vi "Convert_PathWeaverJSON_To_TrajectoryFile.vi"() -> ()   [LabVIEW 2019]
uses:
  <vilib>/Rock Robotics/WPI/ThirdParty/JAS_Junk/TrajLib/TRAJ_STATE.ctl
  <vilib>/Rock Robotics/WPI/ThirdParty/JAS_Junk/TrajLib/POSE2D.ctl
  <vilib>/Rock Robotics/WPI/ThirdParty/JAS_Junk/TrajLib/TRANSLATION2D.ctl
  <vilib>/Rock Robotics/WPI/ThirdParty/JAS_Junk/TrajLib/ROTATION2D.ctl
  <vilib>/Rock Robotics/WPI/ThirdParty/JAS_Junk/TrajLib/DISPLAY_WAYPOINT.ctl
  <vilib>/Rock Robotics/WPI/ThirdParty/JAS_Junk/TrajLib/Trajectory_Library.lvlib
panel:
  in  "End Program":bool
  in  "Tab Control":T1(tab)
  in  "Convert upper left \norigin to lower left":bool
  in  "PathWeaver JSON File":path
  in  "Read JSON Fiile":bool
  out "File Read Error":errorcluster
  in  "PathWeaver Length Units":T2(radio)
  in  "WheelBase":dbl=0.6
  out "Position":cluster{dbl[], dbl[]}[](graph)
  out "Trajectory Data":cluster{dbl[], dbl[]}[](graph)
  out "Traj States\nSize":i32
  out "Trajectory States":T3[](array[typedef]) {"POSE"."ROTATION"."SIN" format="%13.4f"; "POSE"."ROTATION"."COS" format="%13.4f"; "POSE"."ROTATION"."VALUE" format="%13.4f"; "POSE"."TRANSLATION"."Y" format="%14.3f"; "POSE"."TRANSLATION"."X" format="%14.3f"}
  out "File Saved\nWithout\nError":bool
  in  "Trajectory Type":enum32{"Radio Selection 1", "Radio Selection 2"}(radio)
  out "File Creation\nError":errorcluster
  in  "Trajectory File Comment":string
  in  "Trajectory File Name":path
  in  "CreateCmdList":bool
  out "Ready to\nWrite FIle":bool
  # "Convert Pathweaver JSON file to trajectory file"
  # "Instructions: \n---------------- \nThis utility reads a JSON file create from PathWeaver.  The results are plotted for review.  This file can then be written to a Trajectory Library CSV file.\n\nNotes:\n---------\n - Pathweaver sets the Y orign at the top left.  This trajectory library utilties use the bottom right.  This utility converts the Y position value to be consistent. \n   There are no consequences when the trajectory is saved as a robot relative trajectory.  For absolute trajectories, the robot position needs to\n   condier this."
  # "Meters"
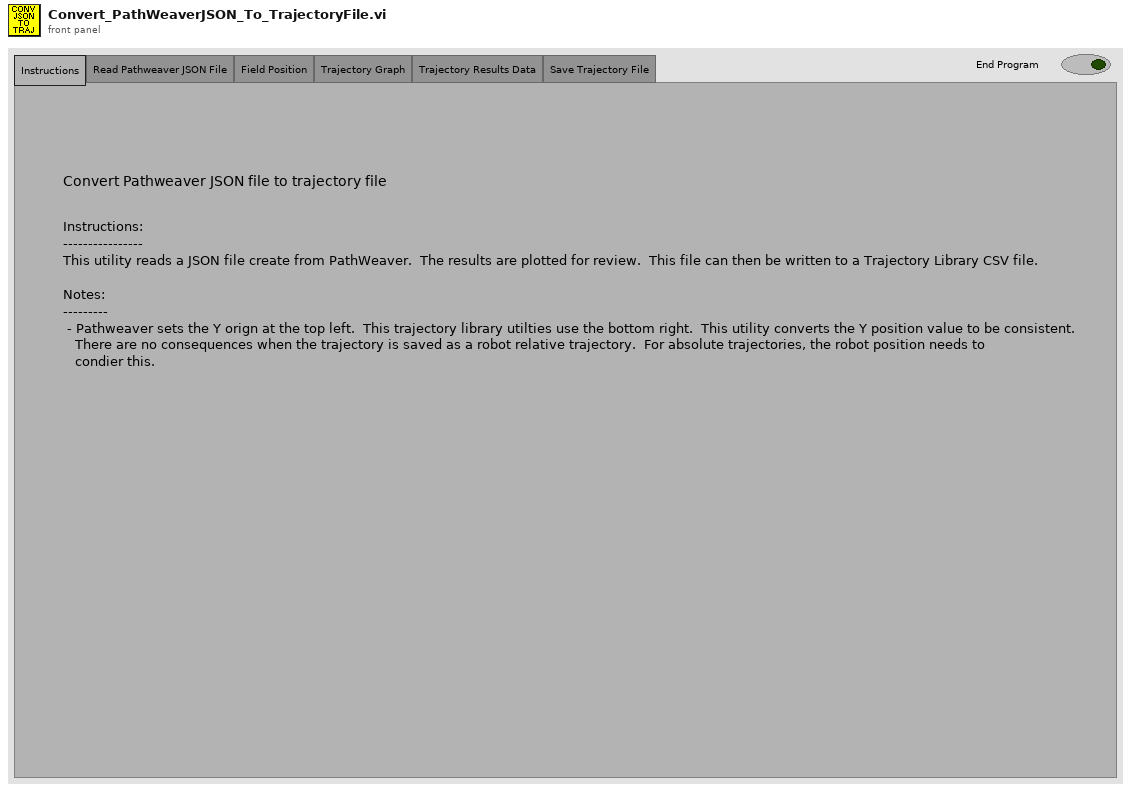
[diagram p1: front panel]
types:
  T1 = enum32{"Instructions", "Read Pathweaver JSON File", "Field Position", "Trajectory Graph", "Trajectory Results Data", "Save Trajectory File"}
  T2 = enum32{"Radio Selection 1", "Radio Selection 2", "Radio Selection 3", "Radio Selection 4", "Radio Selection 5"}
  T3 = typedef "Trajectory_Library.lvlib/TRAJ_STATE.ctl" = cluster{"TimeSeconds":dbl, "Velocity":dbl, "Acceleration":dbl, "POSE":T4, "Curvature":dbl}
  T4 = typedef "Trajectory_Library.lvlib/POSE2D.ctl" = cluster{"TRANSLATION":T5, "ROTATION":T6}
  T5 = typedef "Trajectory_Library.lvlib/TRANSLATION2D.ctl" = cluster{"X":dbl, "Y":dbl}
  T6 = typedef "Trajectory_Library.lvlib/ROTATION2D.ctl" = cluster{"VALUE":dbl, "COS":dbl, "SIN":dbl}
  T7 = typedef "Trajectory_Library.lvlib/DISPLAY_WAYPOINT.ctl" = cluster{"X":dbl, "Y":dbl, "ANGLE":dbl}
  T8 = typedef "Trajectory_Library.lvlib/TRAJECTORY.ctl" = cluster{"TotalTImeSecs":dbl, "States":T3[]}
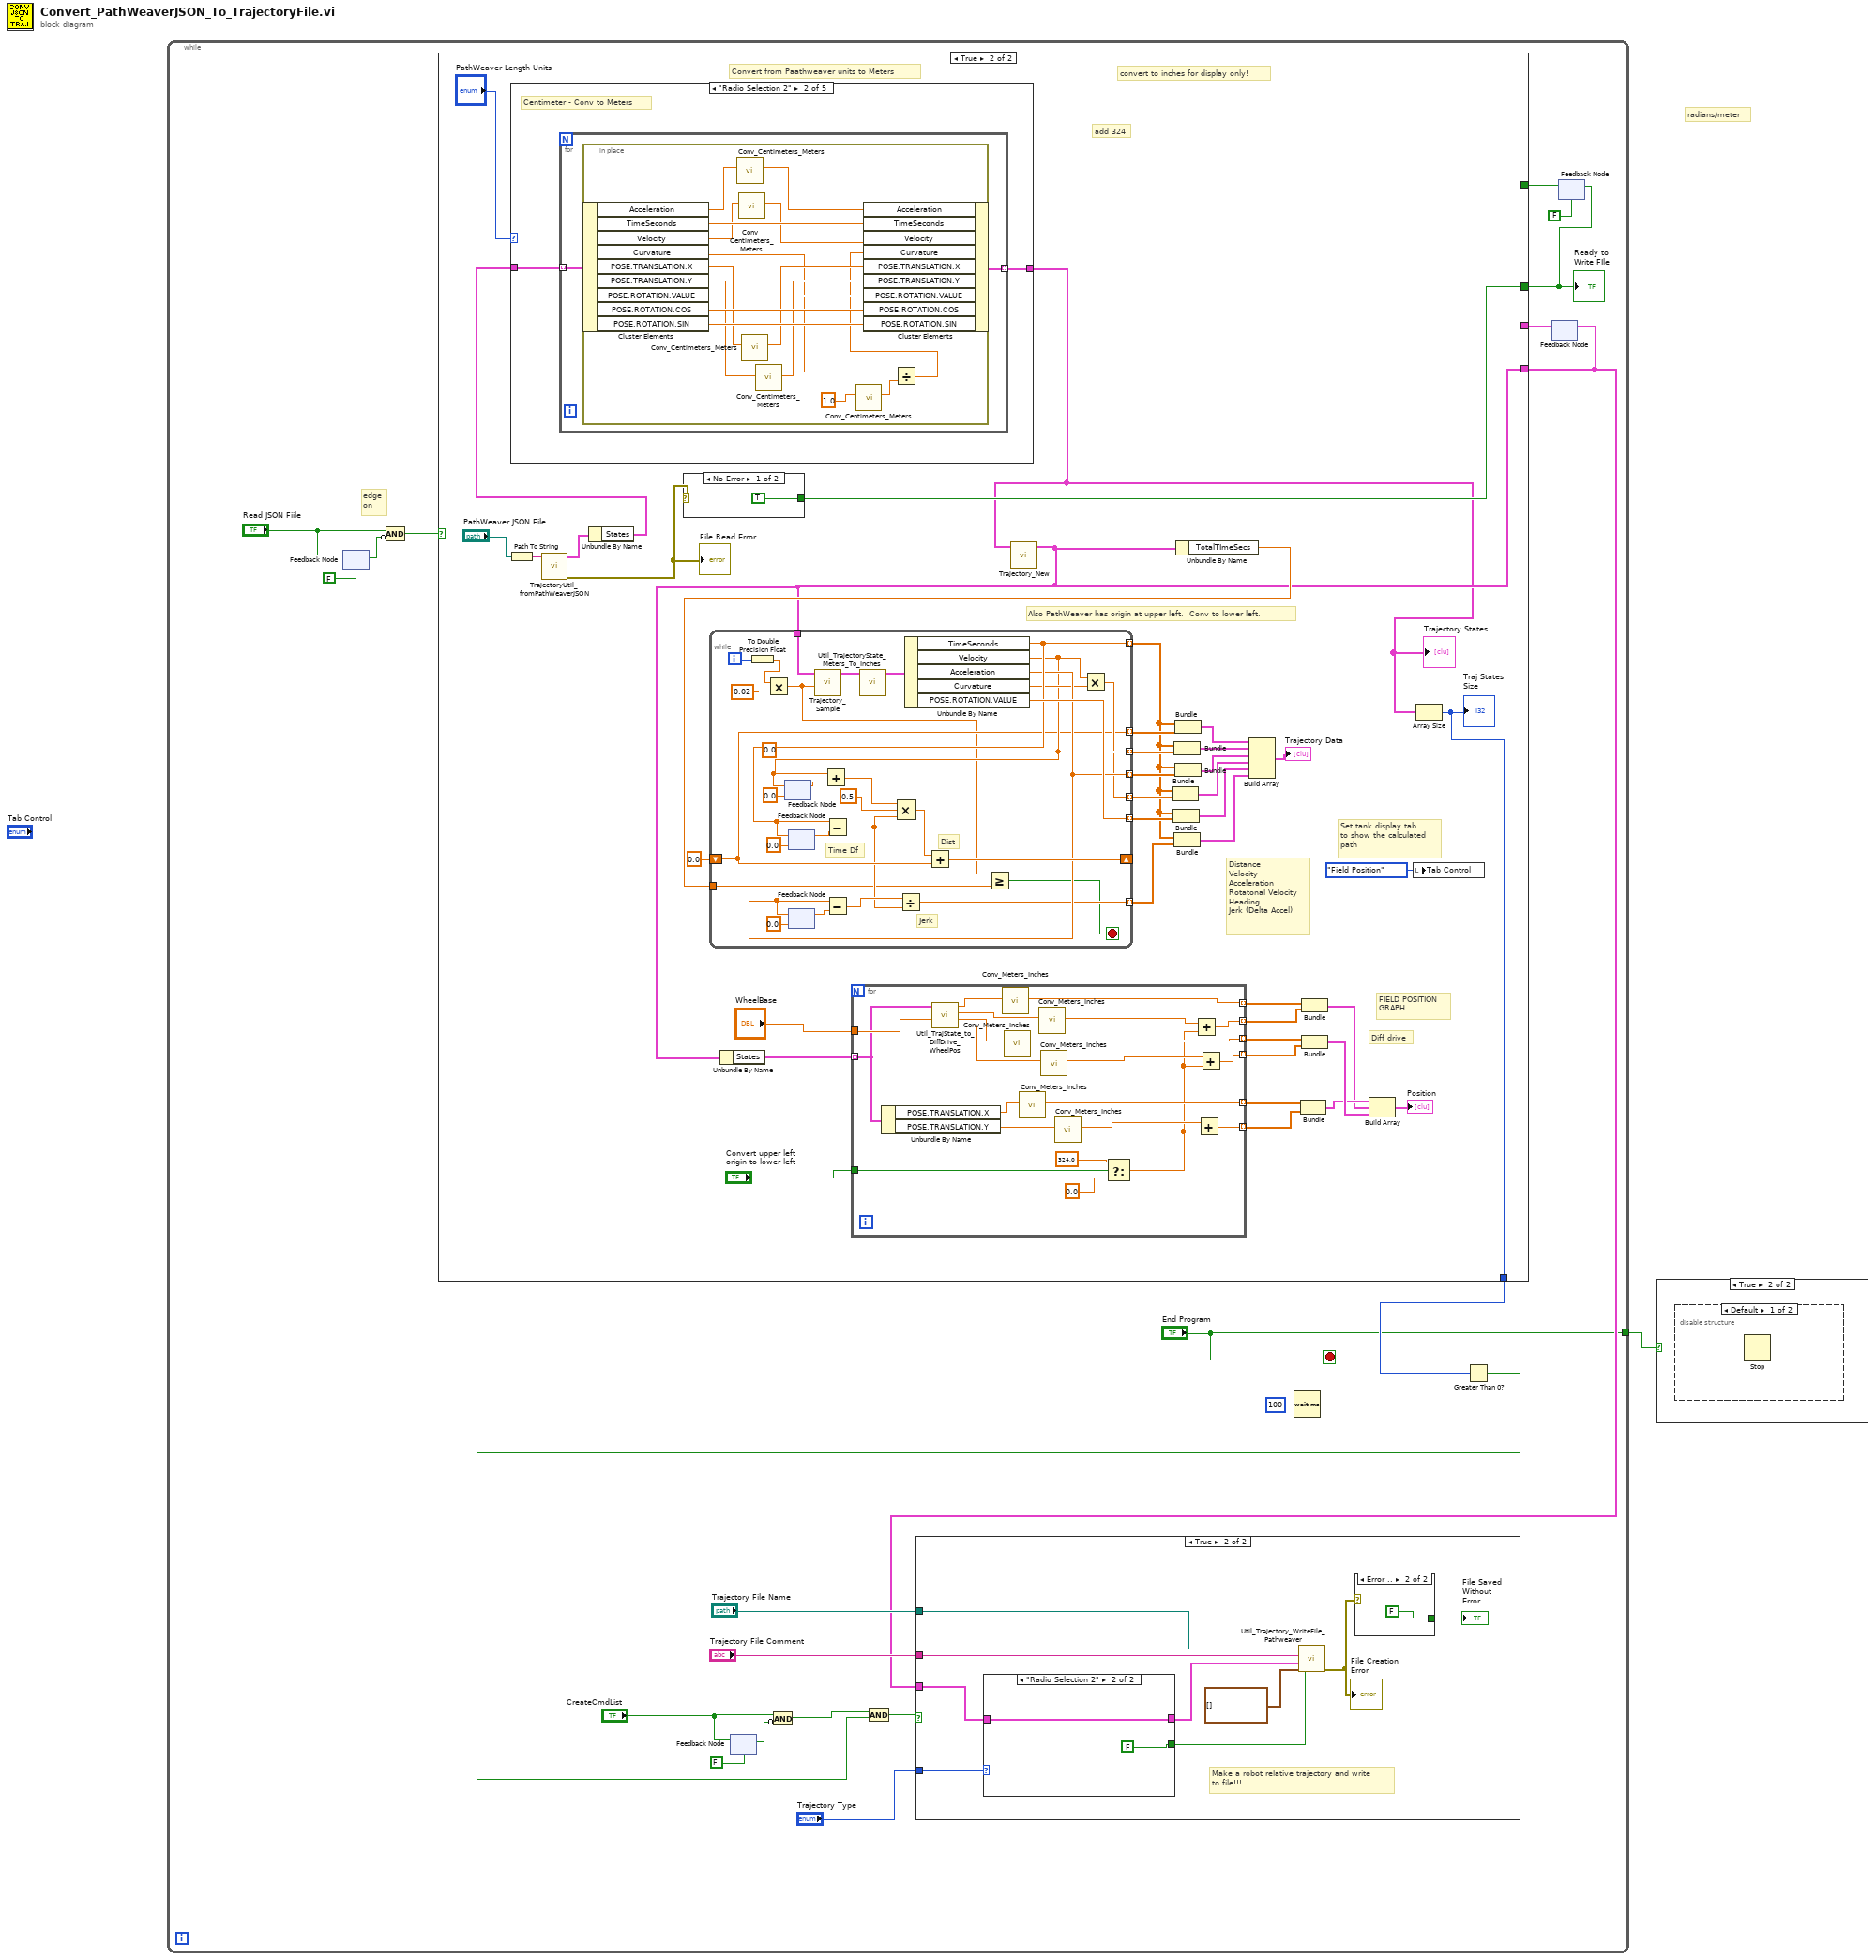
[diagram p0: block diagram]
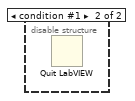
[diagram p3: hidden frame]
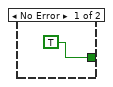
[diagram p5: hidden frame]
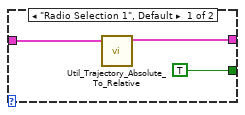
[diagram p6: hidden frame]
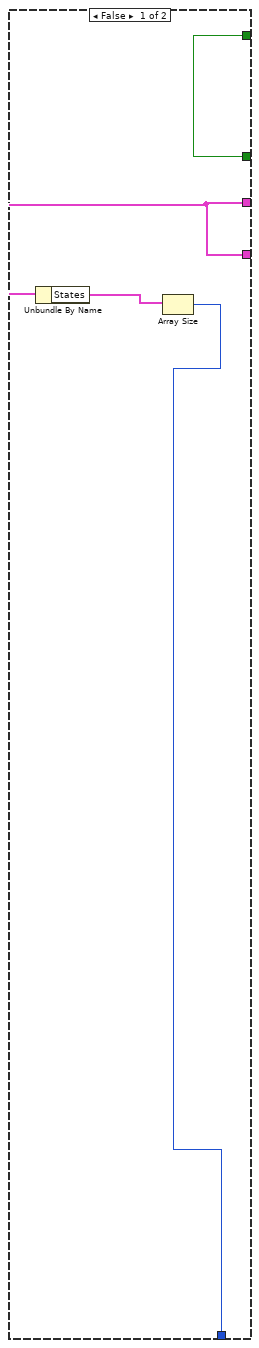
[diagram p7: hidden frame]
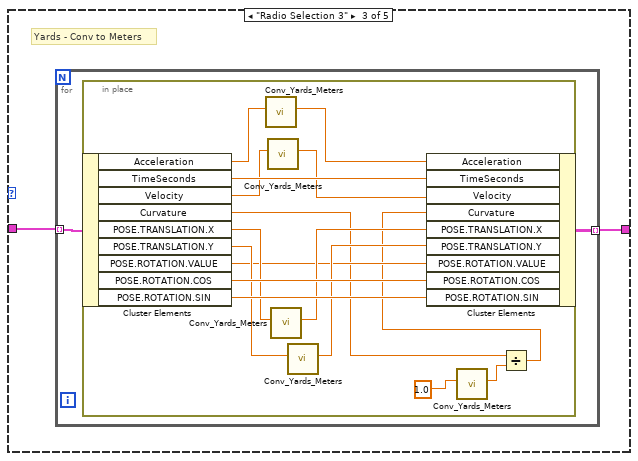
[diagram p9: hidden frame]
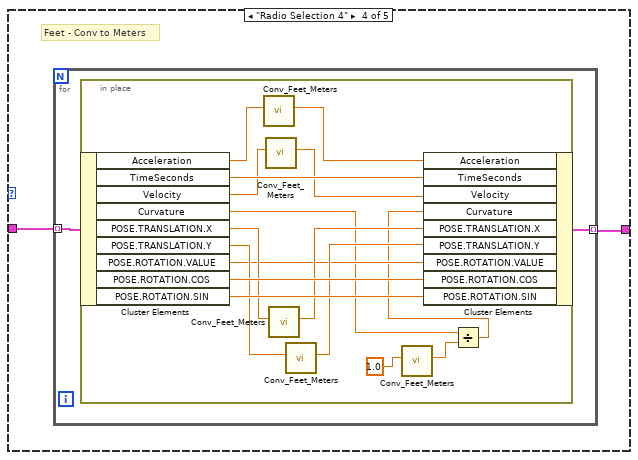
[diagram p10: hidden frame]
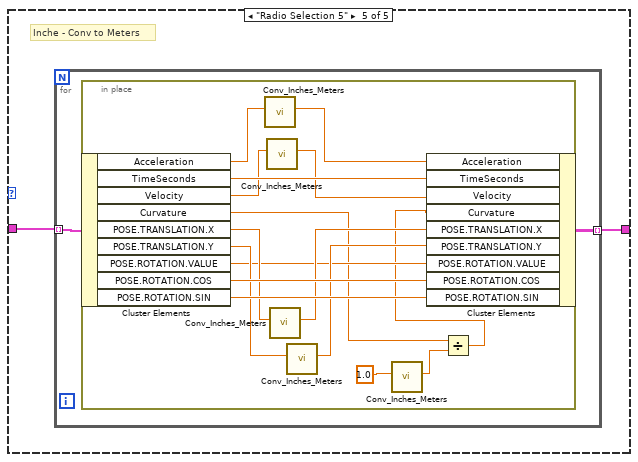
[diagram p11: hidden frame]
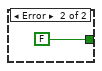
[diagram p12: hidden frame]
diagram:
  # "radians/meter"
  n1 = while {
    tunnel: ["End Program"] -> w1
    stop <- "End Program" stop-if-true
    # "edge\non"
    n2 = feedback #1(FALSE ("CreateCmdList")) -> (w11:bool)
    n3 = feedback-in #1("Read JSON Fiile") -> ()
    n4 = Compound Arithmetic op=AND("Read JSON Fiile", invert w11) -> (w9:bool)
    n5 = feedback-in #2("CreateCmdList") -> ()
    n6 = feedback #2(FALSE ("CreateCmdList")) -> (w14:bool)
    n7 = Compound Arithmetic op=AND("CreateCmdList", invert w14) -> (w13:bool)
    n8 = Wait (ms)(milliseconds to wait=u32 100) -> ()  [unwired: 1 out]
    n9 = feedback #3() -> (w21:T8)  [unwired: 1 in]
    n10 = feedback #4(FALSE) -> (w5:bool)
    n11 = case shown="True" w9 {
      tunnel: [w40 w47] -> w17
      tunnel: w21 -> [w40 _]
      tunnel: [w42 w82] -> w16
      tunnel: [w41 w78] -> w7
      tunnel: w5 -> [w41 _]
      frame False {
        n12 = Unbundle By Name(w40) -> ("States"=w39:T3[])
        n13 = Array Size(array=w39) -> (size(s)=w42:i32)
      }
      frame True {
        (unwired) 0.0
        # "add 324"
        # "Diff drive"
        # "FIELD POSITION\nGRAPH"
        # "Distance\nVelocity\nAcceleration\nRotatonal Velocity\nHeading\nJerk (Delta Accel)"
        # "Also PathWeaver has origin at upper left.  Conv to lower left."
        # "convert to inches for display only!"
        # "Convert from Paathweaver units to Meters"
        # "Set tank display tab\nto show the calculated\npath"
        n14 = Path To String(path="PathWeaver JSON File") -> (string=w81:string)
        n15 = call <vilib>:"TrajectoryUtil_fromPathWeaverJSON.vi"("FileName"=w81) -> ("error out"=w79:errorcluster, "outTRAJECTORY"=w76:T8)  [unwired: 8 in, 1 out]
        "File Read Error" <- w79
        n16 = Unbundle By Name(w76) -> ("States"=w75:T3[])
        n17 = case shown="\"Radio Selection 2\"" "PathWeaver Length Units" {
          tunnel: w75 -> [w133 w134 w155 w175 w195]
          tunnel: [w133 w135 w154 w174 w194] -> w44
          frame "Radio Selection 1" {
            # "Meters - do nothing"
          }
          frame "Radio Selection 2" {
            # "Centimeter - Conv to Meters"
            n18 = for {
              tunnel: w134 -> [w137] mode=indexing
              tunnel: [w136] -> w135 mode=indexing
              n19 = in-place {
                n20 = in-place-cluster #5(w137) -> ("Acceleration"=w145:dbl, "TimeSeconds"=w153:dbl, "Velocity"=w147:dbl, "Curvature"=w138:dbl, "POSE.TRANSLATION.X"=w149:dbl, "POSE.TRANSLATION.Y"=w150:dbl, "POSE.ROTATION.VALUE"=w142:dbl, "POSE.ROTATION.COS"=w152:dbl, "POSE.ROTATION.SIN"=w151:dbl)
                n21 = call <vilib>:"Conv_Centimeters_Meters.vi"("Centimeter"=w145) -> ("Meters"=w144:dbl)  [unwired: 10 in]
                n22 = call <vilib>:"Conv_Centimeters_Meters.vi"("Centimeter"=w147) -> ("Meters"=w146:dbl)  [unwired: 10 in]
                n23 = call <vilib>:"Conv_Centimeters_Meters.vi"("Centimeter"=w149) -> ("Meters"=w148:dbl)  [unwired: 10 in]
                n24 = call <vilib>:"Conv_Centimeters_Meters.vi"("Centimeter"=w150) -> ("Meters"=w143:dbl)  [unwired: 10 in]
                n25 = call <vilib>:"Conv_Centimeters_Meters.vi"("Centimeter"=1.0) -> ("Meters"=w139:dbl)  [unwired: 10 in]
                n26 = Divide(x=w138, y=w139) -> (x/y=w141:dbl)
                n27 = in-place-cluster #5("Acceleration"=w144, "TimeSeconds"=w153, "Velocity"=w146, "Curvature"=w141, "POSE.TRANSLATION.X"=w148, "POSE.TRANSLATION.Y"=w143, "POSE.ROTATION.VALUE"=w142, "POSE.ROTATION.COS"=w152, "POSE.ROTATION.SIN"=w151) -> (w136:T3)
              }
            }
          }
          frame "Radio Selection 3" {
            # "Yards - Conv to Meters"
            n28 = for {
              tunnel: w155 -> [w157] mode=indexing
              tunnel: [w156] -> w154 mode=indexing
              n29 = in-place {
                n30 = in-place-cluster #6(w157) -> ("Acceleration"=w165:dbl, "TimeSeconds"=w173:dbl, "Velocity"=w167:dbl, "Curvature"=w161:dbl, "POSE.TRANSLATION.X"=w169:dbl, "POSE.TRANSLATION.Y"=w170:dbl, "POSE.ROTATION.VALUE"=w162:dbl, "POSE.ROTATION.COS"=w172:dbl, "POSE.ROTATION.SIN"=w171:dbl)
                n31 = call <vilib>:"Conv_Yards_Meters.vi"("Yards"=w165) -> ("Meters"=w164:dbl)  [unwired: 10 in]
                n32 = call <vilib>:"Conv_Yards_Meters.vi"("Yards"=w167) -> ("Meters"=w166:dbl)  [unwired: 10 in]
                n33 = call <vilib>:"Conv_Yards_Meters.vi"("Yards"=w169) -> ("Meters"=w168:dbl)  [unwired: 10 in]
                n34 = call <vilib>:"Conv_Yards_Meters.vi"("Yards"=w170) -> ("Meters"=w163:dbl)  [unwired: 10 in]
                n35 = call <vilib>:"Conv_Yards_Meters.vi"("Yards"=1.0 ("Centimeter")) -> ("Meters"=w159:dbl)  [unwired: 10 in]
                n36 = Divide(x=w161, y=w159) -> (x/y=w160:dbl)
                n37 = in-place-cluster #6("Acceleration"=w164, "TimeSeconds"=w173, "Velocity"=w166, "Curvature"=w160, "POSE.TRANSLATION.X"=w168, "POSE.TRANSLATION.Y"=w163, "POSE.ROTATION.VALUE"=w162, "POSE.ROTATION.COS"=w172, "POSE.ROTATION.SIN"=w171) -> (w156:T3)
              }
            }
          }
          frame "Radio Selection 4" {
            # "Feet - Conv to Meters"
            n38 = for {
              tunnel: w175 -> [w177] mode=indexing
              tunnel: [w176] -> w174 mode=indexing
              n39 = in-place {
                n40 = in-place-cluster #7(w177) -> ("Acceleration"=w185:dbl, "TimeSeconds"=w193:dbl, "Velocity"=w187:dbl, "Curvature"=w179:dbl, "POSE.TRANSLATION.X"=w189:dbl, "POSE.TRANSLATION.Y"=w190:dbl, "POSE.ROTATION.VALUE"=w182:dbl, "POSE.ROTATION.COS"=w192:dbl, "POSE.ROTATION.SIN"=w191:dbl)
                n41 = call <vilib>:"Conv_Feet_Meters.vi"("Feet"=w185) -> ("Meters"=w184:dbl)  [unwired: 10 in]
                n42 = call <vilib>:"Conv_Feet_Meters.vi"("Feet"=w187) -> ("Meters"=w186:dbl)  [unwired: 10 in]
                n43 = call <vilib>:"Conv_Feet_Meters.vi"("Feet"=w189) -> ("Meters"=w188:dbl)  [unwired: 10 in]
                n44 = call <vilib>:"Conv_Feet_Meters.vi"("Feet"=w190) -> ("Meters"=w183:dbl)  [unwired: 10 in]
                n45 = call <vilib>:"Conv_Feet_Meters.vi"("Feet"=1.0 ("Centimeter")) -> ("Meters"=w180:dbl)  [unwired: 10 in]
                n46 = Divide(x=w179, y=w180) -> (x/y=w178:dbl)
                n47 = in-place-cluster #7("Acceleration"=w184, "TimeSeconds"=w193, "Velocity"=w186, "Curvature"=w178, "POSE.TRANSLATION.X"=w188, "POSE.TRANSLATION.Y"=w183, "POSE.ROTATION.VALUE"=w182, "POSE.ROTATION.COS"=w192, "POSE.ROTATION.SIN"=w191) -> (w176:T3)
              }
            }
          }
          frame "Radio Selection 5" {
            # "Inche - Conv to Meters"
            n48 = for {
              tunnel: w195 -> [w197] mode=indexing
              tunnel: [w196] -> w194 mode=indexing
              n49 = in-place {
                n50 = in-place-cluster #8(w197) -> ("Acceleration"=w205:dbl, "TimeSeconds"=w213:dbl, "Velocity"=w207:dbl, "Curvature"=w199:dbl, "POSE.TRANSLATION.X"=w209:dbl, "POSE.TRANSLATION.Y"=w210:dbl, "POSE.ROTATION.VALUE"=w202:dbl, "POSE.ROTATION.COS"=w212:dbl, "POSE.ROTATION.SIN"=w211:dbl)
                n51 = call <vilib>:"Conv_Inches_Meters.vi"("INCH"=w205) -> ("Meters"=w204:dbl)  [unwired: 10 in]
                n52 = call <vilib>:"Conv_Inches_Meters.vi"("INCH"=w207) -> ("Meters"=w206:dbl)  [unwired: 10 in]
                n53 = call <vilib>:"Conv_Inches_Meters.vi"("INCH"=w209) -> ("Meters"=w208:dbl)  [unwired: 10 in]
                n54 = call <vilib>:"Conv_Inches_Meters.vi"("INCH"=w210) -> ("Meters"=w203:dbl)  [unwired: 10 in]
                n55 = call <vilib>:"Conv_Inches_Meters.vi"("INCH"=1.0 ("Centimeter")) -> ("Meters"=w200:dbl)  [unwired: 10 in]
                n56 = Divide(x=w199, y=w200) -> (x/y=w198:dbl)
                n57 = in-place-cluster #8("Acceleration"=w204, "TimeSeconds"=w213, "Velocity"=w206, "Curvature"=w198, "POSE.TRANSLATION.X"=w208, "POSE.TRANSLATION.Y"=w203, "POSE.ROTATION.VALUE"=w202, "POSE.ROTATION.COS"=w212, "POSE.ROTATION.SIN"=w211) -> (w196:T3)
              }
            }
          }
        }
        "Trajectory States" <- w44
        n58 = case shown="No Error" w79 {
          tunnel: [TRUE FALSE] -> w78
          frame No Error {
          }
          frame Error {
          }
        }
        n59 = call <vilib>:"Trajectory_New.vi"("TRAJ_STATES"=w44) -> ("TRAJECTORY"=w47:T8)  [unwired: 10 in]
        n60 = Unbundle By Name(w47) -> ("States"=w46:T3[])
        n61 = for {
          tunnel: w46 -> [w98] mode=indexing
          tunnel: "WheelBase" -> [w103]
          tunnel: [w93] -> w56 mode=indexing
          tunnel: [w95] -> w55 mode=indexing
          tunnel: [w91] -> w54 mode=indexing
          tunnel: [w94] -> w53 mode=indexing
          tunnel: [w88] -> w49 mode=indexing
          tunnel: [w89] -> w48 mode=indexing
          tunnel: "Convert upper left \norigin to lower left" -> [w84]
          n62 = Unbundle By Name(w98) -> ("POSE.TRANSLATION.X"=w97:dbl, "POSE.TRANSLATION.Y"=w96:dbl)
          n63 = call <vilib>:"Util_TrajState_to_DiffDrive_WheelPos.vi"("Wheelbase"=w103, "TRAJ_STATE"=w98) -> ("Right Y"=w99:dbl, "Right X"=w100:dbl, "Left Y"=w101:dbl, "Left X"=w102:dbl)  [unwired: 6 in]
          n64 = call <vilib>:"Conv_Meters_Inches.vi"("Meters"=w102) -> ("Inches"=w93:dbl)  [unwired: 10 in]
          n65 = call <vilib>:"Conv_Meters_Inches.vi"("Meters"=w100) -> ("Inches"=w91:dbl)  [unwired: 10 in]
          n66 = call <vilib>:"Conv_Meters_Inches.vi"("Meters"=w97) -> ("Inches"=w89:dbl)  [unwired: 10 in]
          n67 = call <vilib>:"Conv_Meters_Inches.vi"("Meters"=w101) -> ("Inches"=w92:dbl)  [unwired: 10 in]
          n68 = call <vilib>:"Conv_Meters_Inches.vi"("Meters"=w99) -> ("Inches"=w90:dbl)  [unwired: 10 in]
          n69 = call <vilib>:"Conv_Meters_Inches.vi"("Meters"=w96) -> ("Inches"=w87:dbl)  [unwired: 10 in]
          n70 = Select(t=324.0 ("y"), s=w84, f=0.0) -> (s? t:f=w83:dbl)
          n71 = Add(x=w92, y=w83) -> (x+y=w95:dbl)
          n72 = Add(x=w87, y=w83) -> (x+y=w88:dbl)
          n73 = Add(x=w90, y=w83) -> (x+y=w94:dbl)
        }
        n74 = Unbundle By Name(w47) -> ("TotalTImeSecs"=w59:dbl)
        n75 = while {
          tunnel: [w125] -> w61 mode=indexing
          tunnel: [w116] -> w71 mode=indexing
          tunnel: [w118] -> w70 mode=indexing
          tunnel: [w122] -> w69 mode=indexing
          tunnel: [w117] -> w68 mode=indexing
          tunnel: [w132] -> w67 mode=indexing
          shift-right: [w126] -> _
          shift-left: 0.0 -> [w116]
          tunnel: [w120] -> w60 mode=indexing
          tunnel: w59 -> [w112]
          tunnel: w47 -> [w110]
          i -> [w109]
          stop <- w111 stop-if-true
          # "Time Df"
          # "Jerk"
          # "Dist"
          n76 = To Double Precision Float(number=w109) -> (double precision float=w108:dbl)
          n77 = Multiply(x=w108, y=0.02) -> (x*y=w106:dbl)
          n78 = feedback #9(0.0 ("TimeSeconds")) -> (w128:dbl)
          n79 = feedback #10(0.0 ("TimeSeconds")) -> (w130:dbl)
          n80 = feedback #11(0.0 ("TimeSeconds")) -> (w123:dbl)
          n81 = call <vilib>:"Trajectory_Sample.vi"("Time"=w106, "InputTRAJECTORY"=w110) -> ("OutputTRAJ_STATE"=w104:T3)  [unwired: 9 in]
          n82 = call <vilib>:"Util_TrajectoryState_Meters_To_Inches.vi"("absTRAJECTORY"=w104) -> ("outputRelativeTRAJECTORY"=w105:T3)  [unwired: 10 in]
          n83 = Unbundle By Name(w105) -> ("TimeSeconds"=w125:dbl, "Velocity"=w118:dbl, "Acceleration"=w122:dbl, "Curvature"=w119:dbl, "POSE.ROTATION.VALUE"=w132:dbl)
          n84 = feedback-in #9(w118) -> ()
          n85 = feedback-in #10(w125) -> ()
          n86 = feedback-in #11(w122) -> ()
          n87 = Add(x=w118, y=w128) -> (x+y=w127:dbl)
          n88 = Subtract(x=w125, y=w130) -> (x-y=w113:dbl)
          n89 = Subtract(x=w122, y=w123) -> (x-y=w121:dbl)
          n90 = Compound Arithmetic op=MULTIPLY(w127, 0.5 ("value"), w113) -> (w115:dbl)
          n91 = Divide(x=w121, y=w113) -> (x/y=w120:dbl)
          n92 = Add(x=w115, y=w116) -> (x+y=w126:dbl)
          n93 = Greater Or Equal?(x=w106, y=w112) -> (x >= y?=w111:bool)
          n94 = Multiply(x=w118, y=w119) -> (x*y=w117:dbl)
        }
        n95 = Bundle(w61, w68) -> (w66:cluster{dbl[], dbl[]})  [unwired: 1 in]
        n96 = Bundle(w61, w67) -> (w65:cluster{dbl[], dbl[]})  [unwired: 1 in]
        n97 = Bundle(w61, w70) -> (w73:cluster{dbl[], dbl[]})  [unwired: 1 in]
        n98 = Bundle(w61, w60) -> (w62:cluster{dbl[], dbl[]})  [unwired: 1 in]
        n99 = Bundle(w61, w71) -> (w74:cluster{dbl[], dbl[]})  [unwired: 1 in]
        n100 = Bundle(w61, w69) -> (w72:cluster{dbl[], dbl[]})  [unwired: 1 in]
        n101 = Build Array(w74, w73, w72, w66, w65, w62) -> (→"Trajectory Data":cluster{dbl[], dbl[]}[])
        n102 = Bundle(w48, w49) -> (w51:cluster{dbl[], dbl[]})  [unwired: 1 in]
        n103 = Bundle(w56, w55) -> (w50:cluster{dbl[], dbl[]})  [unwired: 1 in]
        n104 = Bundle(w54, w53) -> (w52:cluster{dbl[], dbl[]})  [unwired: 1 in]
        n105 = Build Array(w51, w50, w52) -> (→"Position":cluster{dbl[], dbl[]}[])
        n106 = local write "Tab Control"(T1."Field Position" ("Tab Control")) -> ()
        n107 = Array Size(array=w44) -> (size(s)=w82:i32)
        "Traj States\nSize" <- w82
      }
    }
    "Ready to\nWrite FIle" <- w7
    n108 = Greater Than 0?(x=w16) -> (x > 0?=w4:bool)
    n109 = And(x=w13, y=w4) -> (x .and. y?=w18:bool)
    n110 = case shown="True" w18 {
      tunnel: "Trajectory File Name" -> [_ w31]
      tunnel: "Trajectory File Comment" -> [_ w30]
      tunnel: w17 -> [_ w27]
      tunnel: "Trajectory Type" -> [_ w28]
      frame False {
      }
      frame True {
        # "Make a robot relative trajectory and write\nto file!!!"
        n111 = case shown="\"Radio Selection 2\"" w28 {
          tunnel: w27 -> [w36 w38]
          tunnel: [w35 w38] -> w26
          tunnel: [TRUE FALSE] -> w23
          frame "Radio Selection 1", Default {
            n112 = call <vilib>:"Util_Trajectory_Absolute_To_Relative.vi"("absTRAJECTORY"=w36) -> ("outputRelativeTRAJECTORY"=w35:T8)  [unwired: 10 in]
          }
          frame "Radio Selection 2" {
          }
        }
        n113 = call <vilib>:"Util_Trajectory_WriteFile_Pathweaver.vi"("Trajectory Is Relative"=w23, "UtilityWayPoints"=T7[] [], "TRAJECTORY"=w26, "Comment"=w30, "Trajectory File Name"=w31) -> ("error out"=w25:errorcluster)  [unwired: 6 in]
        "File Creation\nError" <- w25
        n114 = case shown="Error .." w25 {
          tunnel: [TRUE ("File Saved\nWithout\nError") FALSE ("File Saved\nWithout\nError")] -> w24
          frame No Error {
          }
          frame Error {
          }
        }
        "File Saved\nWithout\nError" <- w24
      }
    }
    n115 = feedback-in #3(w17) -> ()
    n116 = feedback-in #4(w7) -> ()
  }
  n117 = case shown="True" w1 {
    frame False {
    }
    frame True {
      n118 = disable-structure shown="Default" {
        frame condition #0 (active) {
          n119 = Stop() -> ()  [unwired: 1 in]
        }
        frame condition #1 {
          n120 = Quit LabVIEW() -> ()  [unwired: 1 in]
        }
      }
    }
  }
